vi "Query-save-images.vi"(8 "error in":errorcluster, 11 "Storage params. ref. in":refnum<data-value>) -> (0 "error IO":errorcluster, 2 "Save images?":bool, 3 "Storage params. ref.":refnum<data-value>)   [LabVIEW 2013, in "CameraVision.lvlib" / "CV-Storage.lvclass"]
doc: "This function increases the layer/iteration number by one (+1)."
uses:
  CV-Storage.lvclass
  CV-Storage.lvclass/CV-Storage.ctl
  Read Save what.vi
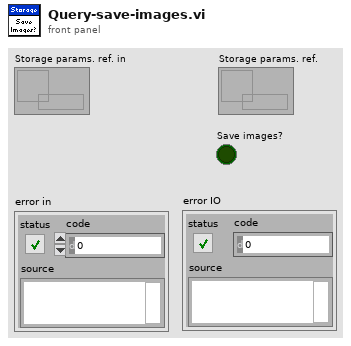
[diagram p1: front panel]
types:
  T1 = cluster{"Original":bool, "Corrected":bool, "Binary":bool, "Temperature":bool, "Characteristics":bool, "Mapping":bool, "TemperatureValues":bool}
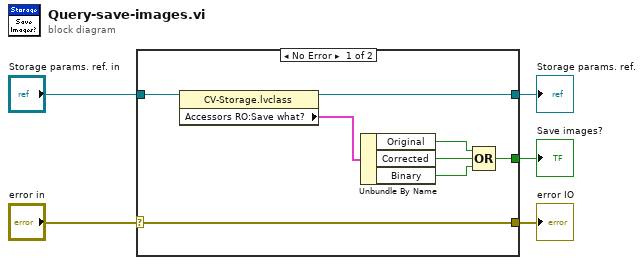
[diagram p0: block diagram]
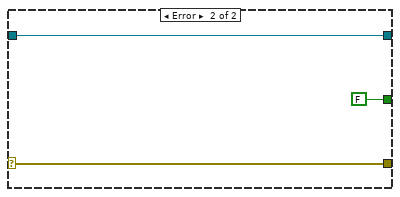
[diagram p2: hidden frame]
diagram:
  n1 = case shown="No Error" "error in" {
    selector: "error in" -> [w6 w16]
    tunnel: [w6 w16] -> w4
    tunnel: "Storage params. ref. in" -> [w13 w15]
    tunnel: [w12 w15] -> w2
    tunnel: [w7 FALSE] -> w1
    frame No Error {
      n2 = property class="CV-Storage.lvclass"(reference=w13) -> (reference out=w12:refnum<data-value>, "Accessors RO:Save what?"=w11:T1)  [unwired: 1 in, 1 out]
      n3 = Unbundle By Name(w11) -> ("Original"=w10:bool, "Corrected"=w9:bool, "Binary"=w8:bool)
      n4 = Compound Arithmetic op=OR(w10, w9, w8) -> (w7:bool)
    }
    frame Error {
    }
  }
  "error IO" <- w4
  "Storage params. ref." <- w2
  "Save images?" <- w1
